vi "ControlPosition.vi"(5 "Control in":refnum<class "Control.lvclass">, 6 "error in":errorcluster, 9 "PythonConverter_GUI in":refnum<class "PythonConverter_GUI.lvclass">) -> (0 "error out":errorcluster, 2 "position":T1, 3 "PythonConverter_GUI out":refnum<class "PythonConverter_GUI.lvclass">, 4 "Control out":refnum<class "Control.lvclass">)   [LabVIEW 2014, in "PythonConverter_GUI.lvclass"]
uses:
  PythonConverter_GUI.lvclass
  VI Interpreter/Classes/Control/Control.lvclass
  <vilib>/Utility/miscctls.llb/LVPositionTypeDef.ctl
  PythonConverter_GUI.lvclass/PythonConverter_GUI.ctl
  VI Interpreter/Classes/GObject/GObject.lvclass/GObject.ctl
  VI Interpreter/Classes/VI Interpreter/VI Interpreter.lvclass
  VI Interpreter/Classes/GObject/GObject.lvclass
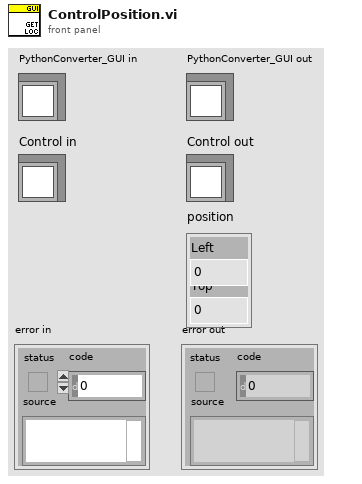
[diagram p1: front panel]
types:
  T1 = typedef "LVPositionTypeDef.ctl" = cluster{"Left":i32, "Top":i32}
  T2 = typedef "PythonConverter_GUI.lvclass/FPOwnerClassTD.ctl" = enum16{"Panel", "Array", "Cluster", "Tab control"}
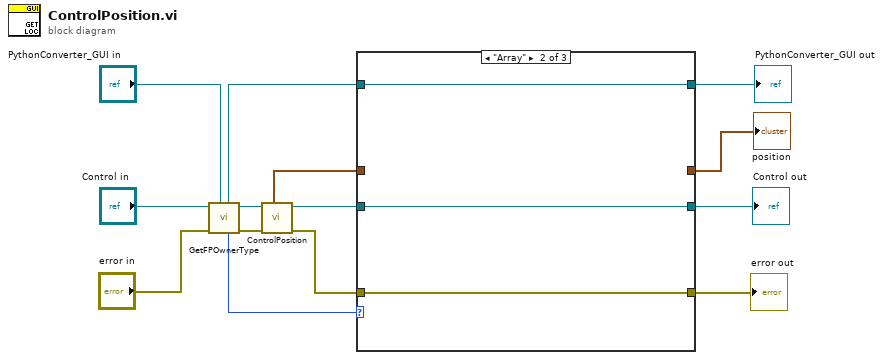
[diagram p0: block diagram]
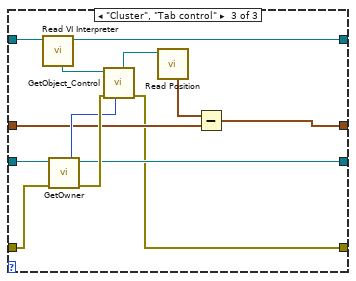
[diagram p3: hidden frame]
diagram:
  n1 = call "GetFPOwnerType.vi"("PythonConverter_GUI in"="PythonConverter_GUI in", "error in"="error in", "Object in"="Control in") -> ("error out"=w4:errorcluster, "Object out"=w5:refnum<class "Control.lvclass">, "owner"=w12:T2, "PythonConverter_GUI out"=w11:refnum<class "PythonConverter_GUI.lvclass">)  [unwired: 5 in]
  n2 = call-dynamic "ControlPosition.vi"("error in"=w4, "Control in"=w5) -> ("error out"=w1:errorcluster, "Control out"=w2:refnum<class "Control.lvclass">, "Position"=w3:T1)  [unwired: 5 in]
  n3 = case shown="\"Array\"" w12 {
    tunnel: w11 -> [w15 w21 w32]
    tunnel: w1 -> [w17 w19 w33]
    tunnel: w2 -> [w16 w20 w34]
    tunnel: w3 -> [w18 _ w28]
    tunnel: [w18 _ w27] -> w9
    tunnel: [w15 w21 w26] -> w10
    tunnel: [w16 w20 w25] -> w6
    tunnel: [w17 w19 w24] -> w8
    frame "Panel" {
    }
    frame "Array" {
    }
    frame "Cluster", "Tab control" {
      n4 = call "Read VI Interpreter.vi"("PythonConverter_GUI in"=w32) -> ("PythonConverter_GUI out"=w26:refnum<class "PythonConverter_GUI.lvclass">, "VI Interpreter"=w31:refnum<class "VI Interpreter.lvclass">)  [unwired: 7 in]
      n5 = call-dynamic "GetOwner.vi"("error in"=w33, "Control in"=w34) -> ("error out"=w30:errorcluster, "Control out"=w25:refnum<class "Control.lvclass">, "Owner"=w29:i32)  [unwired: 5 in]
      n6 = call "GetObject_Control.vi"("UID"=w29, "error in"=w30, "VI Interpreter in"=w31) -> ("error out"=w24:errorcluster, "control"=w23:refnum<class "Control.lvclass">)  [unwired: 3 in, 2 out]
      n7 = call "Read Position.vi"("GObject in"=w23) -> ("Position"=w22:T1)  [unwired: 7 in, 1 out]
      n8 = Subtract(x=w22, y=w28) -> (x-y=w27:T1)
    }
  }
  "error out" <- w8
  "PythonConverter_GUI out" <- w10
  "position" <- w9
  "Control out" <- w6
